vi "Read Publish request data (JSON).vi"(8 "error in (no error)":errorcluster, 11 "Publish JSON in":refnum<class "Publish JSON.lvclass">) -> (0 "error out":errorcluster, 2 "Publish request data (JSON)":T1, 3 "Publish JSON out":refnum<class "Publish JSON.lvclass">)   [LabVIEW 2020, in "wamplv.lvlib" / "Publish JSON.lvclass"]
uses:
  Publish JSON.lvclass
  Publish JSON.lvclass/Publish JSON.ctl
  WAMP Client/API/TypeDefs/Error or abort detail (JSON).ctl
  wamplv.lvlib
  WAMP Client/API/TypeDefs/Combined error.ctl
  WAMP Client/Private/TypeDef/PUBLISH result (JSON).ctl
  WAMP Client/Private/TypeDef/PUBLISH Request Data (JSON).ctl
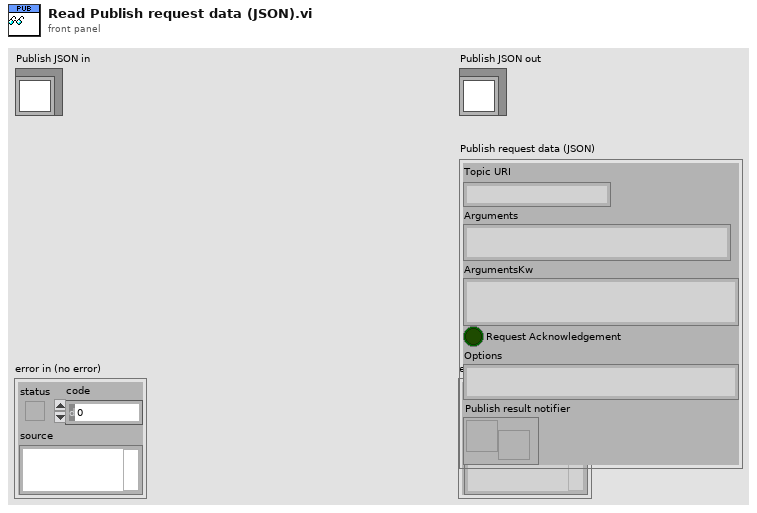
[diagram p1: front panel]
types:
  T1 = typedef "wamplv.lvlib/PUBLISH Request Data (JSON).ctl" = cluster{"Topic URI":string, "Arguments":string, "ArgumentsKw":string, "Request Acknowledgement":bool, "Options":string, "Publish result notifier":refnum<notifier>}
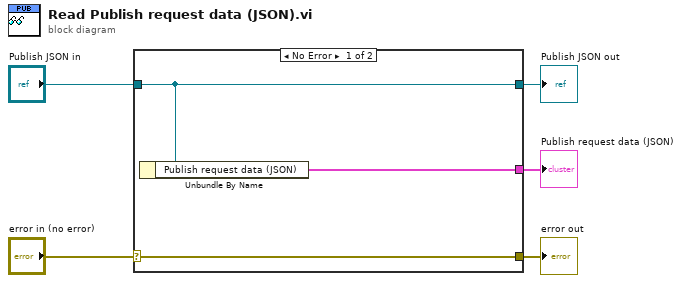
[diagram p0: block diagram]
diagram:
  n1 = case shown="No Error" "error in (no error)" {
    selector: "error in (no error)" -> [w8 w9]
    tunnel: [w8 w9] -> w4
    tunnel: [w7 w10] -> w2
    tunnel: "Publish JSON in" -> [w7 w10]
    tunnel: [w6 _] -> w1
    frame No Error {
      n2 = Unbundle By Name(w7) -> ("Publish request data (JSON)"=w6:T1)
    }
    frame Error {
    }
  }
  "error out" <- w4
  "Publish JSON out" <- w2
  "Publish request data (JSON)" <- w1
